vi "Euler(degree_Step).vi"(8 "Offset":dbl min=-5.0 max=5.0 step=0.01, 9 "Max Field for Triangle":dbl=1.05 min=-9.0 max=9.0 step=0.01, 10 "Ring":u16(ring) items=["Constant Field Sweep", "R - trangle wave"], 11 "Cluster":T1={"R1"=1.99, "R2"=1.99, "theta 1 (deg)"=0.0, "theta 2 (deg)"=360.0, "phi 1 (deg)"=90.0, "phi 2 (deg)"=90.0, "Step Size (T/deg/deg)"=2.5, "Stepping Parameter"=enum."Theta"} {"phi 2 (deg)" format="%#_13g"; "phi 1 (deg)" format="%#_13g"; "theta 2 (deg)" format="%#_13g"; "theta 1 (deg)" format="%#_13g"; "R2" min=-2.0 max=2.0 step=0.01 format="%#_13g"; "R1" min=-2.0 max=2.0 step=0.01 format="%#_13g"}) -> (3 "Waveform Graph":dbl[][](graph)=[[1.99, 1.988105960947897, 1.9824274492025735, 1.9729752741338826, 1.9597674284942939, 1.9428290541686675, 1.922192394315246, 1.8978967319889717, 1.8699883153639578, 1.8385202696974605, 1.8035524962029335, 1.7651515580246613, 1.723390553531033, 1.6783489771676425, 1.6301125681350936, 1.578773147179558, 1.5244284418067662, 1.467181900252147, 1.4071424945612296, 1.3444245131551642, 1.2791473432762133, 1.2114352437273541, 1.1414171083385818, 1.0692262206101795, 0.9950000000000002, 0.9188797403377178, 0.8410103408639918, 0.7615400304065287, 0.6806200852180809, 0.5984045410135038, 0.5150498997540163, 0.4307148317368248, 0.34555987355719153, 0.2597471225179029, 0.17343992806784014, 0.08680258085701865, 1.2185235651516163e-16, -0.08680258085701842, -0.17343992806783945, -0.25974712251790266, -0.3455598735571913, -0.43071483173682457, -0.515049899754016, -0.5984045410135032, -0.6806200852180807, -0.7615400304065285, -0.8410103408639916, -0.9188797403377171, -0.9949999999999996, -1.0692262206101788, -1.1414171083385811, -1.2114352437273541, -1.2791473432762133, -1.344424513155164, -1.4071424945612294, -1.4671819002521467, -1.524428441806766, -1.5787731471795579, -1.6301125681350932, -1.678348977167642, -1.723390553531033, -1.7651515580246613, -1.8035524962029335, -1.8385202696974605, -1.8699883153639576, -1.8978967319889715, -1.9221923943152457, -1.9428290541686672, -1.9597674284942939, -1.9729752741338826, -1.9824274492025735, -1.988105960947897, -1.99, -1.988105960947897, -1.9824274492025735, -1.9729752741338829, -1.959767428494294, -1.9428290541686677, -1.922192394315246, -1.8978967319889717, -1.8699883153639578, -1.8385202696974607, -1.8035524962029337, -1.7651515580246615, -1.7233905535310332, -1.6783489771676428, -1.630112568135094, -1.578773147179558, -1.5244284418067662, -1.467181900252147, -1.4071424945612299, -1.3444245131551642, -1.2791473432762135, -1.2114352437273546, -1.1414171083385822, -1.0692262206101801, -0.9950000000000009, -0.9188797403377185, -0.8410103408639928, -0.7615400304065297, -0.680620085218082, -0.5984045410135032, -0.515049899754016, -0.4307148317368246, -0.34555987355719137, -0.2597471225179027, -0.17343992806783992, -0.0868025808570189, -3.655570695454849e-16, 0.08680258085701817, 0.1734399280678392, 0.259747122517902, 0.34555987355719064, 0.4307148317368239, 0.5150498997540154, 0.5984045410135025, 0.6806200852180796, 0.7615400304065274, 0.8410103408639906, 0.9188797403377178, 0.9950000000000002, 1.0692262206101795, 1.1414171083385816, 1.211435243727354, 1.279147343276213, 1.3444245131551638, 1.4071424945612292, 1.4671819002521465, 1.5244284418067657, 1.5787731471795576, 1.6301125681350932, 1.678348977167642, 1.7233905535310323, 1.7651515580246608, 1.803552496202933, 1.83852026969746, 1.8699883153639572, 1.8978967319889712, 1.922192394315246, 1.9428290541686675, 1.9597674284942939, 1.9729752741338826, 1.9824274492025735, 1.988105960947897], [0.0, 0.08680258085701864, 0.17343992806783975, 0.2597471225179026, 0.34555987355719137, 0.43071483173682473, 0.5150498997540163, 0.5984045410135035, 0.6806200852180807, 0.7615400304065286, 0.8410103408639918, 0.9188797403377175, 0.9949999999999999, 1.0692262206101795, 1.1414171083385816, 1.2114352437273541, 1.279147343276213, 1.3444245131551638, 1.4071424945612294, 1.4671819002521467, 1.5244284418067662, 1.578773147179558, 1.6301125681350936, 1.6783489771676425, 1.7233905535310328, 1.765151558024661, 1.8035524962029335, 1.8385202696974605, 1.8699883153639576, 1.8978967319889715, 1.922192394315246, 1.9428290541686675, 1.9597674284942939, 1.9729752741338826, 1.9824274492025735, 1.988105960947897, 1.99, 1.988105960947897, 1.9824274492025735, 1.9729752741338826, 1.9597674284942939, 1.9428290541686675, 1.922192394315246, 1.8978967319889717, 1.8699883153639578, 1.8385202696974605, 1.8035524962029337, 1.7651515580246615, 1.723390553531033, 1.6783489771676428, 1.630112568135094, 1.578773147179558, 1.5244284418067662, 1.467181900252147, 1.4071424945612296, 1.3444245131551642, 1.2791473432762135, 1.2114352437273546, 1.1414171083385822, 1.06922622061018, 0.9949999999999999, 0.9188797403377175, 0.841010340863992, 0.7615400304065288, 0.680620085218081, 0.5984045410135039, 0.5150498997540168, 0.43071483173682534, 0.3455598735571921, 0.2597471225179026, 0.1734399280678398, 0.08680258085701878, 2.4370471303032327e-16, -0.0868025808570183, -0.1734399280678393, -0.2597471225179021, -0.34555987355719076, -0.430714831736824, -0.5150498997540164, -0.5984045410135034, -0.6806200852180806, -0.7615400304065284, -0.8410103408639915, -0.9188797403377171, -0.9949999999999994, -1.0692262206101788, -1.1414171083385811, -1.2114352437273541, -1.279147343276213, -1.3444245131551638, -1.4071424945612294, -1.4671819002521465, -1.524428441806766, -1.5787731471795576, -1.6301125681350932, -1.678348977167642, -1.7233905535310323, -1.7651515580246608, -1.803552496202933, -1.83852026969746, -1.8699883153639574, -1.8978967319889717, -1.922192394315246, -1.9428290541686675, -1.9597674284942939, -1.9729752741338826, -1.9824274492025735, -1.988105960947897, -1.99, -1.988105960947897, -1.9824274492025735, -1.9729752741338829, -1.959767428494294, -1.9428290541686677, -1.9221923943152461, -1.897896731988972, -1.869988315363958, -1.838520269697461, -1.8035524962029341, -1.765151558024661, -1.7233905535310328, -1.6783489771676425, -1.6301125681350936, -1.578773147179558, -1.5244284418067664, -1.4671819002521471, -1.4071424945612299, -1.3444245131551644, -1.2791473432762137, -1.2114352437273546, -1.1414171083385825, -1.0692262206101801, -0.9950000000000009, -0.9188797403377185, -0.841010340863993, -0.7615400304065298, -0.6806200852180821, -0.5984045410135049, -0.5150498997540162, -0.43071483173682473, -0.3455598735571915, -0.25974712251790283, -0.17343992806784006, -0.08680258085701903], [1.2185235651516163e-16, 1.2185235651516163e-16, 1.2185235651516163e-16, 1.2185235651516163e-16, 1.2185235651516163e-16, 1.2185235651516163e-16, 1.2185235651516163e-16, 1.2185235651516163e-16, 1.2185235651516163e-16, 1.2185235651516163e-16, 1.2185235651516163e-16, 1.2185235651516163e-16, 1.2185235651516163e-16, 1.2185235651516163e-16, 1.2185235651516163e-16, 1.2185235651516163e-16, 1.2185235651516163e-16, 1.2185235651516163e-16, 1.2185235651516163e-16, 1.2185235651516163e-16, 1.2185235651516163e-16, 1.2185235651516163e-16, 1.2185235651516163e-16, 1.2185235651516163e-16, 1.2185235651516163e-16, 1.2185235651516163e-16, 1.2185235651516163e-16, 1.2185235651516163e-16, 1.2185235651516163e-16, 1.2185235651516163e-16, 1.2185235651516163e-16, 1.2185235651516163e-16, 1.2185235651516163e-16, 1.2185235651516163e-16, 1.2185235651516163e-16, 1.2185235651516163e-16, 1.2185235651516163e-16, 1.2185235651516163e-16, 1.2185235651516163e-16, 1.2185235651516163e-16, 1.2185235651516163e-16, 1.2185235651516163e-16, 1.2185235651516163e-16, 1.2185235651516163e-16, 1.2185235651516163e-16, 1.2185235651516163e-16, 1.2185235651516163e-16, 1.2185235651516163e-16, 1.2185235651516163e-16, 1.2185235651516163e-16, 1.2185235651516163e-16, 1.2185235651516163e-16, 1.2185235651516163e-16, 1.2185235651516163e-16, 1.2185235651516163e-16, 1.2185235651516163e-16, 1.2185235651516163e-16, 1.2185235651516163e-16, 1.2185235651516163e-16, 1.2185235651516163e-16, 1.2185235651516163e-16, 1.2185235651516163e-16, 1.2185235651516163e-16, 1.2185235651516163e-16, 1.2185235651516163e-16, 1.2185235651516163e-16, 1.2185235651516163e-16, 1.2185235651516163e-16, 1.2185235651516163e-16, 1.2185235651516163e-16, 1.2185235651516163e-16, 1.2185235651516163e-16, 1.2185235651516163e-16, 1.2185235651516163e-16, 1.2185235651516163e-16, 1.2185235651516163e-16, 1.2185235651516163e-16, 1.2185235651516163e-16, 1.2185235651516163e-16, 1.2185235651516163e-16, 1.2185235651516163e-16, 1.2185235651516163e-16, 1.2185235651516163e-16, 1.2185235651516163e-16, 1.2185235651516163e-16, 1.2185235651516163e-16, 1.2185235651516163e-16, 1.2185235651516163e-16, 1.2185235651516163e-16, 1.2185235651516163e-16, 1.2185235651516163e-16, 1.2185235651516163e-16, 1.2185235651516163e-16, 1.2185235651516163e-16, 1.2185235651516163e-16, 1.2185235651516163e-16, 1.2185235651516163e-16, 1.2185235651516163e-16, 1.2185235651516163e-16, 1.2185235651516163e-16, 1.2185235651516163e-16, 1.2185235651516163e-16, 1.2185235651516163e-16, 1.2185235651516163e-16, 1.2185235651516163e-16, 1.2185235651516163e-16, 1.2185235651516163e-16, 1.2185235651516163e-16, 1.2185235651516163e-16, 1.2185235651516163e-16, 1.2185235651516163e-16, 1.2185235651516163e-16, 1.2185235651516163e-16, 1.2185235651516163e-16, 1.2185235651516163e-16, 1.2185235651516163e-16, 1.2185235651516163e-16, 1.2185235651516163e-16, 1.2185235651516163e-16, 1.2185235651516163e-16, 1.2185235651516163e-16, 1.2185235651516163e-16, 1.2185235651516163e-16, 1.2185235651516163e-16, 1.2185235651516163e-16, 1.2185235651516163e-16, 1.2185235651516163e-16, 1.2185235651516163e-16, 1.2185235651516163e-16, 1.2185235651516163e-16, 1.2185235651516163e-16, 1.2185235651516163e-16, 1.2185235651516163e-16, 1.2185235651516163e-16, 1.2185235651516163e-16, 1.2185235651516163e-16, 1.2185235651516163e-16, 1.2185235651516163e-16, 1.2185235651516163e-16, 1.2185235651516163e-16, 1.2185235651516163e-16, 1.2185235651516163e-16, 1.2185235651516163e-16, 1.2185235651516163e-16]])   [LabVIEW 2013]
uses:
  <vilib>/Native 3D Graph/xcontrol/3DPC_SurfacePlot.xctl
  <vilib>/Native 3D Graph/classes/Line/Line.lvclass
  <vilib>/Analysis/coordinate.llb/3D Coordinate Conversion (Array).vi
  <vilib>/Analysis/coordinate.llb/3D Cartesian Coordinate Rotation (Euler) (Array).vi
  <vilib>/gmath/NI_Gmath.lvlib
  <vilib>/Analysis/NI_AALPro.lvlib
panel:
  out "concatenated string":string="1.050000*(2*(abs(2*((x+(0.250000))/1-floor((x+(0.250000))/1+1/2))))-1)"
  out "Waveform Graph 2":dbl[](graph)=[1.99, 1.99, 1.99, 1.99, 1.9899999999999998, 1.99, 1.99, 1.99, 1.9900000000000002, 1.9899999999999998, 1.99, 1.99, 1.99, 1.99, 1.99, 1.9900000000000002, 1.9899999999999998, 1.99, 1.99, 1.99, 1.99, 1.9900000000000002, 1.99, 1.99, 1.99, 1.99, 1.99, 1.99, 1.99, 1.99, 1.99, 1.99, 1.9899999999999998, 1.99, 1.99, 1.99, 1.99, 1.99, 1.99, 1.99, 1.9899999999999998, 1.99, 1.99, 1.99, 1.9900000000000002, 1.9899999999999998, 1.9900000000000002, 1.9900000000000002, 1.9899999999999998, 1.9899999999999998, 1.99, 1.9900000000000002, 1.99, 1.9900000000000002, 1.99, 1.99, 1.99, 1.9900000000000002, 1.99, 1.9899999999999998, 1.99, 1.99, 1.99, 1.99, 1.99, 1.99, 1.99, 1.99, 1.99, 1.99, 1.99, 1.9900000000000002, 1.99, 1.99, 1.9899999999999998, 1.99, 1.99, 1.9900000000000002, 1.99, 1.99, 1.99, 1.99, 1.99, 1.9900000000000002, 1.99, 1.9899999999999998, 1.99, 1.9900000000000002, 1.9899999999999998, 1.99, 1.99, 1.99, 1.99, 1.99, 1.99, 1.99, 1.99, 1.9900000000000002, 1.99, 1.99, 1.9900000000000002, 1.99, 1.99, 1.99, 1.9899999999999998, 1.99, 1.99, 1.9900000000000002, 1.99, 1.99, 1.9899999999999998, 1.99, 1.99, 1.9900000000000002, 1.99, 1.99, 1.99, 1.9899999999999998, 1.99, 1.99, 1.99, 1.99, 1.99, 1.99, 1.99, 1.9900000000000002, 1.99, 1.99, 1.9899999999999998, 1.99, 1.99, 1.99, 1.99, 1.9900000000000002, 1.99, 1.99, 1.99, 1.9900000000000002, 1.99, 1.99, 1.9899999999999998, 1.99, 1.99, 1.9900000000000002]
  out "After Euler Rotation":refnum<class "Base Datatype.lvclass">[](xcontrol)
  in  "Euler Angles (deg)":cluster{"phi":dbl, "theta":dbl, "psi":dbl}
  out "3D Graph":refnum<class "Base Datatype.lvclass">[](xcontrol) caption="Trace"
  # "Note: (1) R2-R1 = how many triangles\n          (2) 1 extra step is added for the \n                 LabVIEW built-in array gene-\n                  ration function.\n          (3) Offset: as multiples of period\n                (0.5 = shift 1 trangle leftward)"
  # "Phi = Rotation about Z-axis\nTheta = Rotation about X'-axis\nPsi = Rotation about Z'-axis"
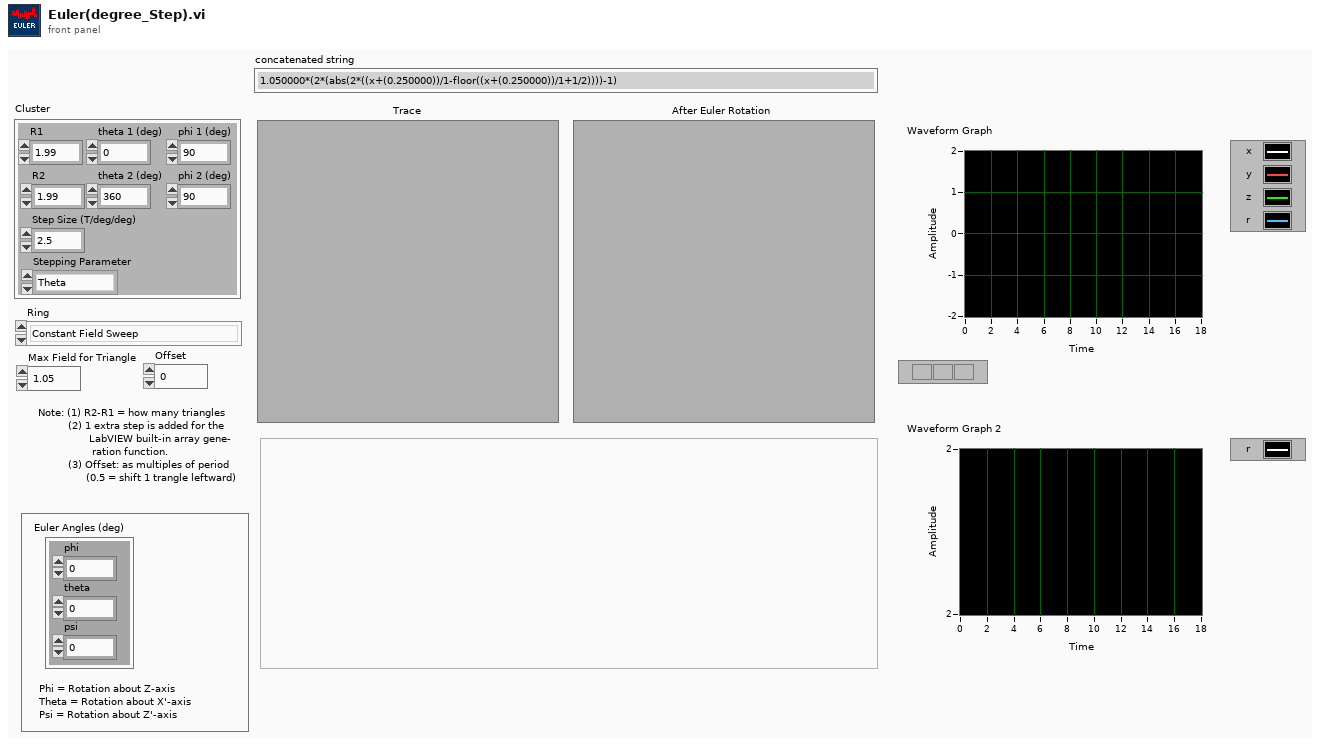
[diagram p1: front panel]
types:
  T1 = cluster{"R1":dbl, "R2":dbl, "theta 1 (deg)":dbl, "theta 2 (deg)":dbl, "phi 1 (deg)":dbl, "phi 2 (deg)":dbl, "Step Size (T/deg/deg)":dbl, "Stepping Parameter":enum16{"R", "Theta", "Phi"}}
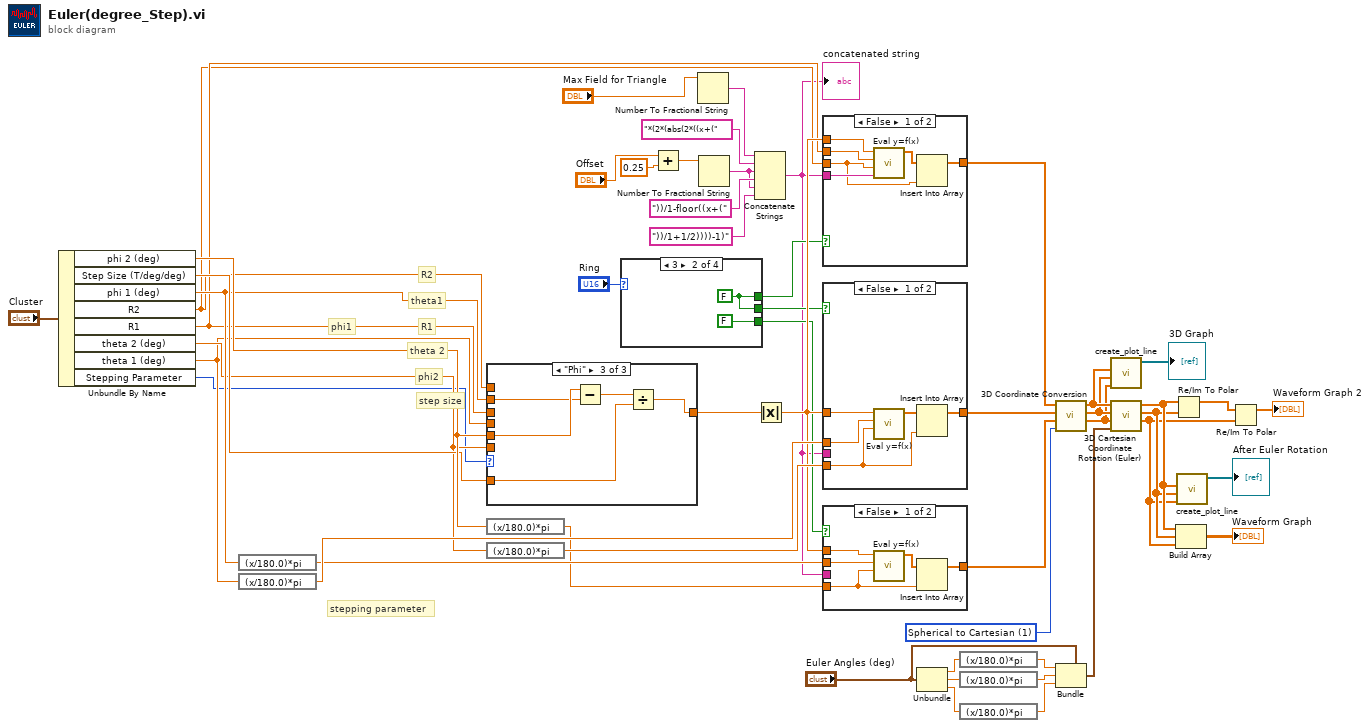
[diagram p0: block diagram]
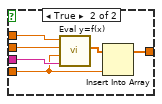
[diagram p2: hidden frame]
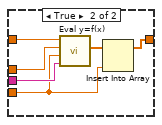
[diagram p3: hidden frame]
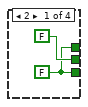
[diagram p4: hidden frame]
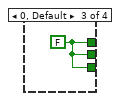
[diagram p5: hidden frame]
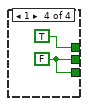
[diagram p6: hidden frame]
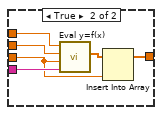
[diagram p7: hidden frame]
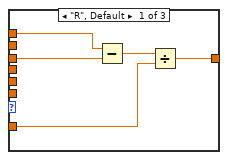
[diagram p8: hidden frame]
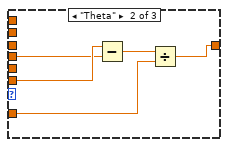
[diagram p9: hidden frame]
diagram:
  w52 = u16 1 items=["Cartesian to Spherical", "Spherical to Cartesian", "Cartesian to Cylindrical", "Cylindrical to Cartesian", "Spherical to Cylindrical", "Cylindrical to Spherical"] ("conversion type")
  # "step size"
  # "stepping parameter"
  # "phi1"
  # "phi2"
  # "R1"
  # "R2"
  # "theta1"
  # "theta 2"
  n1 = Unbundle By Name("Cluster") -> ("phi 2 (deg)"=w31:dbl, "Step Size (T/deg/deg)"=w30:dbl, "phi 1 (deg)"=w29:dbl, "R2"=w18:dbl, "R1"=w19:dbl, "theta 2 (deg)"=w28:dbl, "theta 1 (deg)"=w27:dbl, "Stepping Parameter"=w26:enum16{"R", "Theta", "Phi"})
  n2 = expression code="(x/180.0)*pi" ("degrees to radians")(w29) -> (w46:dbl)
  n3 = expression code="(x/180.0)*pi" ("degrees to radians")(w27) -> (w48:dbl)
  n4 = case shown="\"Phi\"" w26 {
    tunnel: w30 -> [w53 w59 w63]
    tunnel: [w57 w58 w67] -> w1
    tunnel: w31 -> [_ _ w65]
    tunnel: w29 -> [_ _ w64]
    tunnel: w28 -> [_ w62 _]
    tunnel: w27 -> [_ w61 _]
    tunnel: w18 -> [w55 _ _]
    tunnel: w19 -> [w54 _ _]
    frame "R", Default {
      n5 = Subtract(x=w55, y=w54) -> (x-y=w56:dbl)
      n6 = Divide(x=w56, y=w53) -> (x/y=w57:dbl)
    }
    frame "Theta" {
      n7 = Subtract(x=w62, y=w61) -> (x-y=w60:dbl)
      n8 = Divide(x=w60, y=w59) -> (x/y=w58:dbl)
    }
    frame "Phi" {
      n9 = Subtract(x=w65, y=w64) -> (x-y=w66:dbl)
      n10 = Divide(x=w66, y=w63) -> (x/y=w67:dbl)
    }
  }
  n11 = expression code="(x/180.0)*pi" ("degrees to radians")(w31) -> (w45:dbl)
  n12 = expression code="(x/180.0)*pi" ("degrees to radians")(w28) -> (w47:dbl)
  n13 = case shown="3" "Ring" {
    tunnel: [w68 w70 w72 TRUE] -> w14
    tunnel: [FALSE w70 w72 w73] -> w13
    tunnel: [w68 FALSE w72 w73] -> w12
    frame 2 {
      w68 = FALSE
    }
    frame 3 {
      w70 = FALSE
    }
    frame 0, Default {
      w72 = FALSE
    }
    frame 1 {
      w73 = FALSE
    }
  }
  n14 = Add(x="Offset", y=0.25) -> (x+y=w5:dbl)
  n15 = Number To Fractional String(number="Max Field for Triangle") -> (F-format string=w10:string)  [unwired: 3 in]
  n16 = Number To Fractional String(number=w5) -> (F-format string=w7:string)  [unwired: 3 in]
  n17 = Concatenate Strings(w10, "*(2*(abs(2*((x+(" ("string"), w7, "))/1-floor((x+(" ("string"), w7, "))/1+1/2))))-1)" ("string")) -> (w11:string)
  "concatenated string" <- w11
  n18 = Absolute Value(x=w1) -> (abs(x)=w20:dbl)
  n19 = case shown="False" w14 {
    tunnel: w20 -> [w80 w86]
    tunnel: w19 -> [w77 w85]
    tunnel: w18 -> [w75 w82]
    tunnel: [w76 w81] -> w17
    tunnel: w11 -> [w79 w84]
    frame False {
      n20 = call <vilib>:"Eval y=f(x).vi"("formula"=w79, "end"=w75, "start"=w77, "number of points"=w80) -> ("X Values"=w78:dbl[])  [unwired: 3 out]
      n21 = Insert Into Array(array=w78, new element=w75) -> (w76:dbl[])  [unwired: 1 in]
    }
    frame True {
      n22 = call <vilib>:"Eval y=f(x).vi"("formula"=w84, "end"=w82, "start"=w85, "number of points"=w86) -> ("Y Values"=w83:dbl[])  [unwired: 3 out]
      n23 = Insert Into Array(array=w83, new element=w82) -> (w81:dbl[])  [unwired: 1 in]
    }
  }
  n24 = case shown="False" w13 {
    tunnel: [w87 w92] -> w2
    tunnel: w48 -> [w90 w97]
    tunnel: w47 -> [w88 w93]
    tunnel: w20 -> [w91 w96]
    tunnel: w11 -> [_ w95]
    frame False {
      n25 = call <vilib>:"Eval y=f(x).vi"("end"=w88, "start"=w90, "number of points"=w91) -> ("X Values"=w89:dbl[])  [unwired: 1 in, 3 out]
      n26 = Insert Into Array(array=w89, new element=w88) -> (w87:dbl[])  [unwired: 1 in]
    }
    frame True {
      n27 = call <vilib>:"Eval y=f(x).vi"("formula"=w95, "end"=w93, "start"=w97, "number of points"=w96) -> ("Y Values"=w94:dbl[])  [unwired: 3 out]
      n28 = Insert Into Array(array=w94, new element=w93) -> (w92:dbl[])  [unwired: 1 in]
    }
  }
  n29 = case shown="False" w12 {
    tunnel: [w98 w104] -> w50
    tunnel: w46 -> [w101 w108]
    tunnel: w45 -> [w99 w103]
    tunnel: w20 -> [w102 w107]
    tunnel: w11 -> [_ w106]
    frame False {
      n30 = call <vilib>:"Eval y=f(x).vi"("end"=w99, "start"=w101, "number of points"=w102) -> ("X Values"=w100:dbl[])  [unwired: 1 in, 3 out]
      n31 = Insert Into Array(array=w100, new element=w99) -> (w98:dbl[])  [unwired: 1 in]
    }
    frame True {
      n32 = call <vilib>:"Eval y=f(x).vi"("formula"=w106, "end"=w103, "start"=w108, "number of points"=w107) -> ("Y Values"=w105:dbl[])  [unwired: 3 out]
      n33 = Insert Into Array(array=w105, new element=w103) -> (w104:dbl[])  [unwired: 1 in]
    }
  }
  n34 = Unbundle("Euler Angles (deg)") -> ("phi"=w44:dbl, "theta"=w43:dbl, "psi"=w42:dbl)
  n35 = expression code="(x/180.0)*pi" ("degrees to radians")(w44) -> (w41:dbl)
  n36 = expression code="(x/180.0)*pi" ("degrees to radians")(w43) -> (w40:dbl)
  n37 = expression code="(x/180.0)*pi" ("degrees to radians")(w42) -> (w39:dbl)
  n38 = call-poly <vilib>:"3D Coordinate Conversion.vi"("conversion type"=w52, "Axis 3"=w50, "Axis 2"=w2, "Axis 1"=w17) -> ("Axis 3 Out"=w34:dbl[], "Axis 2 Out"=w35:dbl[], "Axis 1 Out"=w36:dbl[])  [unwired: 4 in, 1 out]
  n39 = Bundle(cluster="Euler Angles (deg)", "phi"=w41, "theta"=w40, "psi"=w39) -> (w37:cluster{"phi":dbl, "theta":dbl, "psi":dbl})
  n40 = call <vilib>:"create_plot_line.vi"("z vector"=w34, "y vector"=w35, "x vector"=w36) -> ("plots out"=→"3D Graph":refnum<class "Base Datatype.lvclass">[])  [unwired: 2 in, 6 out]
  n41 = call-poly <vilib>:"3D Cartesian Coordinate Rotation (Euler).vi"("Euler Angles"=w37, "Z"=w34, "Y"=w35, "X"=w36) -> ("Z Out"=w22:dbl[], "Y Out"=w23:dbl[], "X Out"=w24:dbl[])  [unwired: 4 in, 1 out]
  n42 = Re/Im To Polar(2:w23, 3:w24) -> (1:w25:dbl[])  [unwired: 1 out]
  n43 = Build Array(w24, w23, w22) -> (→"Waveform Graph":dbl[][])
  n44 = call <vilib>:"create_plot_line.vi"("z vector"=w22, "y vector"=w23, "x vector"=w24) -> ("plots out"=→"After Euler Rotation":refnum<class "Base Datatype.lvclass">[])  [unwired: 2 in, 6 out]
  n45 = Re/Im To Polar(2:w22, 3:w25) -> (1:→"Waveform Graph 2":dbl[])  [unwired: 1 out]
